vi "PrepareAndSendROI.vi"(8 "error in (no error)":errorcluster, 9 "ROI":T1, 10 "Clear ROI?(F)":bool=TRUE, 11 "CameraController in":refnum<class "CameraController.lvclass">) -> (0 "error out":errorcluster, 3 "CameraController out":refnum<class "CameraController.lvclass">)   [LabVIEW 2020, in "CameraController.lvlib" / "CameraController.lvclass"]
uses:
  CameraController.lvclass
  C:/Program Files/National Instruments/LabVIEW 2020/vi.lib/ActorFramework/Actor/Actor.lvclass
  <vilib>/ActorFramework/Actor/Actor.lvclass/Actor.ctl
  CameraController.lvclass/CameraController.ctl
  <vilib>/ActorFramework/Message Enqueuer/Message Enqueuer.lvclass/Message Enqueuer.ctl
  Model/Hardware Abstraction Layer/Component/Camera/Camera Messages/SetROI Msg/SetROI Msg.lvclass/SetROI Msg.ctl
  <vilib>/ActorFramework/Message Enqueuer/Enqueue.vi
  Model/Hardware Abstraction Layer/Component/Camera/Camera Messages/ClearROI Msg/ClearROI Msg.lvclass
  C:/Program Files/National Instruments/LabVIEW 2020/vi.lib/ActorFramework/Message/Message.lvclass
  Model/Hardware Abstraction Layer/Component/Camera/Camera Messages/SetROI Msg/SetROI Msg.lvclass
  <vilib>/ActorFramework/Message Priority Queue/Priority Enqueue.vi
  <vilib>/ActorFramework/Actor/Actor.lvclass
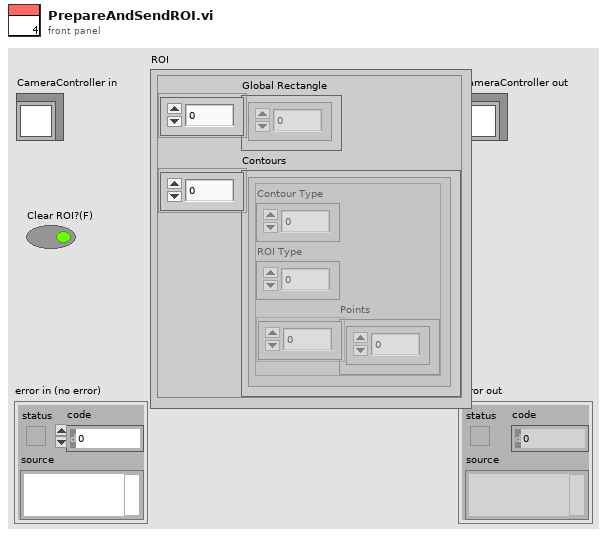
[diagram p1: front panel]
types:
  T1 = cluster{"Global Rectangle":i32[], "Contours":cluster{"Contour Type":u32, "ROI Type":u32, "Points":i32[]}[]}
  T2 = cluster{"x":dbl, "y":dbl, "width":dbl, "height":dbl}
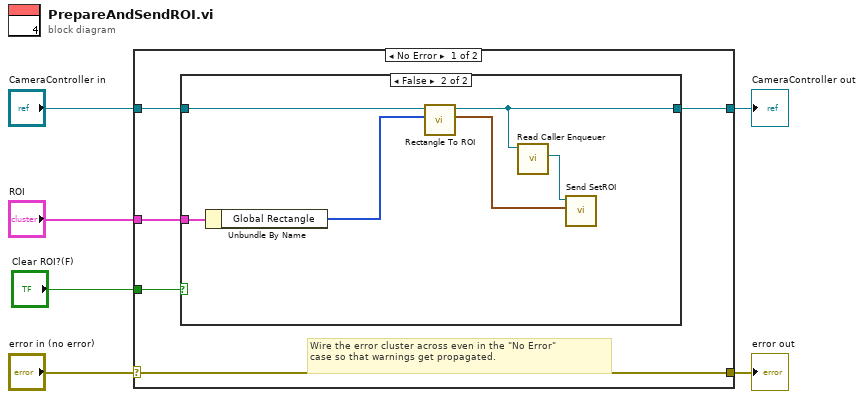
[diagram p0: block diagram]
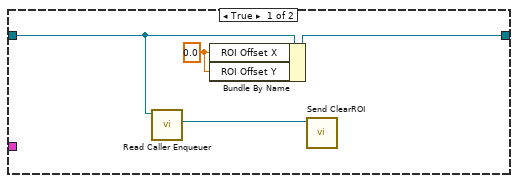
[diagram p2: hidden frame]
diagram:
  n1 = case shown="No Error" "error in (no error)" {
    selector: "error in (no error)" -> [w11 w23]
    tunnel: [w11 w23] -> w5
    tunnel: [w8 w22] -> w3
    tunnel: "CameraController in" -> [w9 w22]
    tunnel: "ROI" -> [w10 _]
    tunnel: "Clear ROI?(F)" -> [w7 _]
    frame No Error {
      # "Wire the error cluster across even in the \"No Error\"\ncase so that warnings get propagated."
      n2 = case shown="False" w7 {
        tunnel: w10 -> [_ w21]
        tunnel: w9 -> [w13 w20]
        tunnel: [w15 w18] -> w8
        frame True {
          w14 = 0.0 ("ROI Offset X")
          n3 = call <vilib>:"Read Caller Enqueuer.vi"("Actor"=w13) -> ("Caller Enqueuer"=w12:refnum<class "Message Enqueuer.lvclass">)  [unwired: 10 in]
          n4 = Bundle By Name(cluster=w13, "ROI Offset X"=w14, "ROI Offset Y"=w14) -> (w15:refnum<class "CameraController.lvclass">)
          n5 = call "Send ClearROI.vi"("Message Enqueuer"=w12) -> ()  [unwired: 9 in, 2 out]
        }
        frame False {
          n6 = Unbundle By Name(w21) -> ("Global Rectangle"=w19:i32[])
          n7 = call-dynamic "Rectangle To ROI.vi"("Global Rectangle in"=w19, "Camera Prime95B Controller in"=w20) -> ("Setting.ROI"=w16:T2, "Camera Prime95B Controller out"=w18:refnum<class "CameraController.lvclass">)  [unwired: 7 in, 1 out]
          n8 = call <vilib>:"Read Caller Enqueuer.vi"("Actor"=w18) -> ("Caller Enqueuer"=w17:refnum<class "Message Enqueuer.lvclass">)  [unwired: 10 in]
          n9 = call "Send SetROI.vi"("Setting.ROI"=w16, "Message Enqueuer"=w17) -> ()  [unwired: 8 in, 2 out]
        }
      }
    }
    frame Error {
    }
  }
  "error out" <- w5
  "CameraController out" <- w3
